vi "Verify_CRC.vi"(5 "CRC32C":string, 7 "CRC32":string, 8 "error in (no error)":errorcluster, 9 "Path to Log File":path, 10 "Path to Project File":string, 11 "Path to JFlash.exe":string) -> (0 "error out":errorcluster, 2 "Pass":bool)   [LabVIEW 2025]
panel:
  # "Example for CRC:\nCRC of data = 0x06A5F442, CRC of file = 0x06A5F442)"
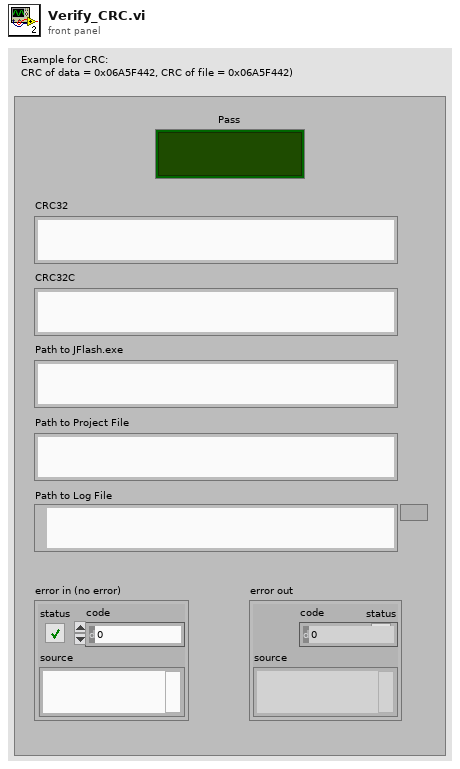
[diagram p1: front panel]
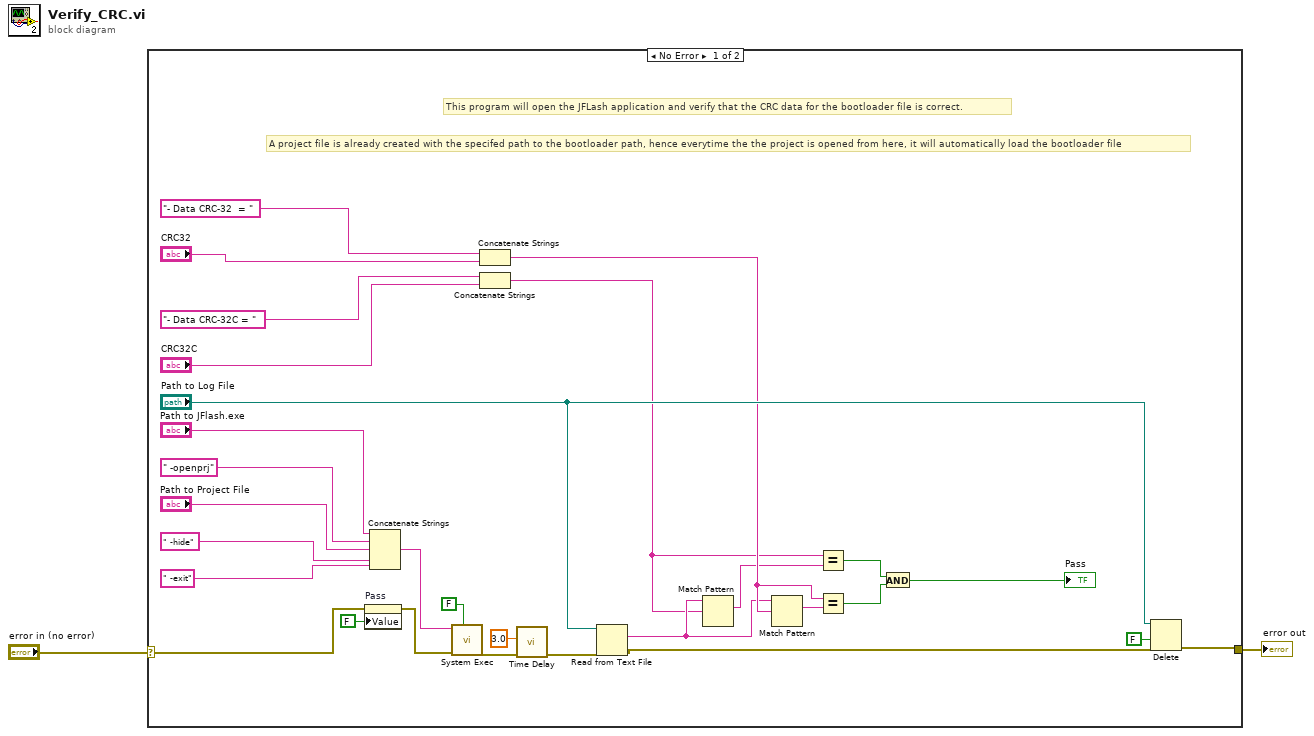
[diagram p0: block diagram]
diagram:
  n1 = case shown="No Error" "error in (no error)" {
    selector: "error in (no error)" -> [w23 w32]
    tunnel: [w19 w32] -> w2
    frame No Error {
      # "A project file is already created with the specifed path to the bootloader path, hence everytime the the project is opened from here, it will automatically load the bootloader file"
      # "This program will open the JFLash application and verify that the CRC data for the bootloader file is correct."
      n2 = property on="Pass" class="Bool (strict)"(error in=w23, "Value"=FALSE ("Pass")) -> (error out=w24:errorcluster)  [unwired: 1 in, 1 out]
      n3 = Concatenate Strings("Path to JFlash.exe", " -openprj" ("string"), "Path to Project File", " -hide" ("string"), " -exit" ("string")) -> (w26:string)
      n4 = call <vilib>:"System Exec.vi"("wait until completion? (T)"=FALSE, "error in (no error)"=w24, "command line"=w26) -> ("error out"=w16:errorcluster)  [unwired: 5 in, 3 out]
      n5 = Concatenate Strings("- Data CRC-32  = " ("string"), "CRC32") -> (w11:string)
      n6 = Concatenate Strings("- Data CRC-32C = " ("string"), "CRC32C") -> (w6:string)
      n7 = call "Time Delay"("error in (no error)"=w16, "Delay Time (s)"=3.0) -> ("error out"=w17:errorcluster)  [unwired: 9 in]
      n8 = Read from Text File(file (use dialog)="Path to Log File", error in=w17) -> (text=w8:string, error out=w20:errorcluster)  [unwired: 2 in, 2 out]
      n9 = Match Pattern(string=w8, regular expression=w6) -> (match substring=w7:string)  [unwired: 1 in, 3 out]
      n10 = Match Pattern(string=w8, regular expression=w11) -> (match substring=w12:string)  [unwired: 1 in, 3 out]
      n11 = Equal?(x=w6, y=w7) -> (x = y?=w5:bool)
      n12 = Equal?(x=w11, y=w12) -> (x = y?=w4:bool)
      n13 = And(x=w5, y=w4) -> (x .and. y?=→"Pass":bool)
      n14 = Delete(path (use dialog)="Path to Log File", confirm (F)=FALSE, error in=w20) -> (error out=w19:errorcluster)  [unwired: 2 in, 2 out]
    }
    frame Error {
    }
  }
  "error out" <- w2
